vi "Init Communication.vi"(8 "error in (no error)":errorcluster, 10 "Voltage Length":u32, 11 "Item Ref in":T2 format="%.0x") -> (0 "error out":errorcluster, 2 "Communication":T1, 3 "Item Ref out":T2 format="%.0x")   [LabVIEW 2011, in "Switch-DMM Custom Device.lvlib"]
uses:
  Switch-DMM Custom Device.lvlib
  <vilib>/NI Veristand/Custom Device API/Custom Device Item Ref.ctl
  Controls/Communication.ctl
  Controls/Async Status.ctl
  Controls/Async State.ctl
  Controls/Async Command.ctl
  Controls/Async Events.ctl
  <vilib>/NI Veristand/Custom Device API/Custom Device API.lvlib
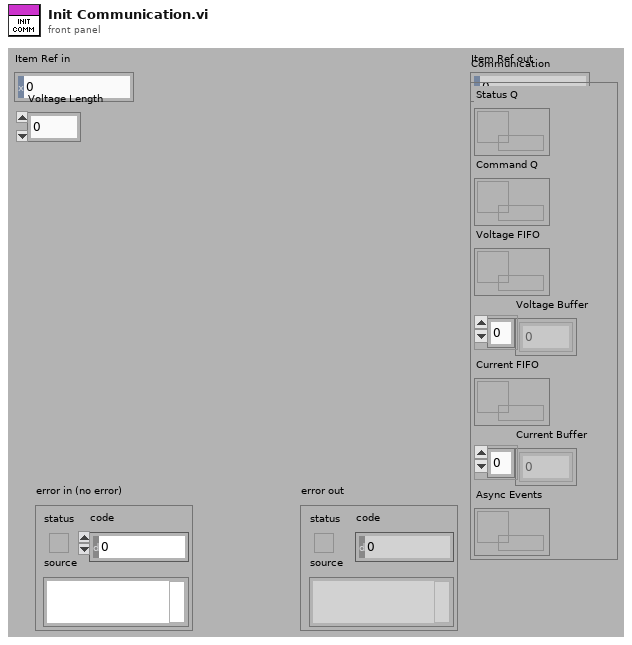
[diagram p1: front panel]
types:
  T1 = typedef "Switch-DMM Custom Device.lvlib/Communication.ctl" = cluster{"Status Q":refnum<queue>, "Command Q":refnum<queue>, "Voltage FIFO":refnum<k33>, "Voltage Buffer":dbl[], "Current FIFO":refnum<k33>, "Current Buffer":dbl[], "Async Events":refnum<queue>}
  T2 = typedef "Custom Device API.lvlib/Custom Device Item Ref.ctl" = u64
  T3 = typedef "Switch-DMM Custom Device.lvlib/Async Events.ctl" = enum16{"None", "Over Current", "Volt Read Done"}
  T4 = typedef "Switch-DMM Custom Device.lvlib/Async Status.ctl" = cluster{"State":T5, "error":errorcluster}
  T5 = typedef "Switch-DMM Custom Device.lvlib/Async State.ctl" = enum16{"Not running", "Initializing", "Waiting on start cmd", "Running", "Stopped"}
  T6 = typedef "Switch-DMM Custom Device.lvlib/Async Command.ctl" = enum16{"None", "Start", "Set Cur Mode", "Req Volt Mode", "Set Volt Mode", "Read Volt", "Exit"}
  T7 = cluster{"read mode":enum16{"polling", "blocking"}, "write mode":enum16{"polling", "blocking"}}
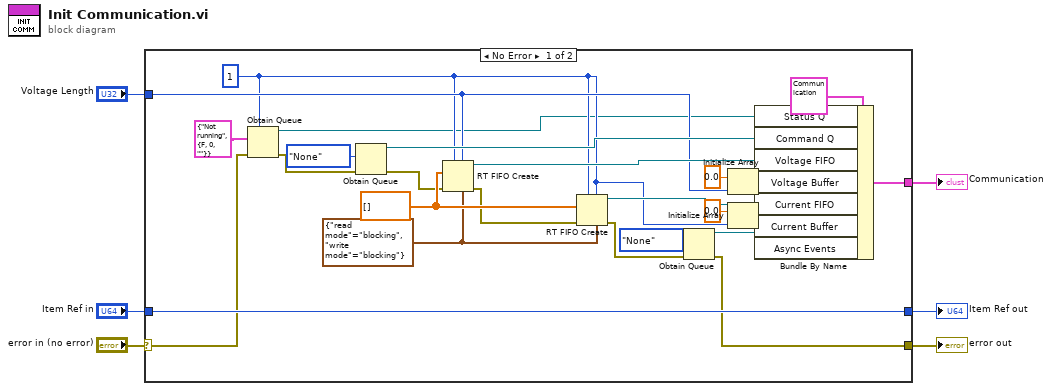
[diagram p0: block diagram]
diagram:
  n1 = case shown="No Error" "error in (no error)" {
    selector: "error in (no error)" -> [w16 w33]
    tunnel: "Item Ref in" -> [w19 w32]
    tunnel: [w7 w33] -> w4
    tunnel: [w19 w32] -> w3
    tunnel: "Voltage Length" -> [w18 _]
    tunnel: [w13 _] -> w1
    frame No Error {
      w24 = T7 {"read mode"=enum."blocking", "write mode"=enum."blocking"} ("r/w modes (polling,polling)")
      w25 = dbl[] []
      w12 = u32 1 ("size (10)")
      n2 = Obtain Queue(max queue size (-1, unlimited)=w12, element data type=T4 {"State"=enum."Not running", "error"={"status"=FALSE, "code"=0, "source"=""}} ("Async Status"), error in (no error)=w16) -> (queue out=w11:refnum<queue>, error out=w17:errorcluster)  [unwired: 2 in, 1 out]
      n3 = Obtain Queue(element data type=Async_Command."None" ("Async Command"), error in (no error)=w17) -> (queue out=w28:refnum<queue>, error out=w15:errorcluster)  [unwired: 3 in, 1 out]
      n4 = RT FIFO Create(1:w25, 3:w15, 4:w12, 6:w18, 7:w24) -> (8:w23:refnum<k33>, 11:w14:errorcluster)  [unwired: 3 in, 1 out]
      n5 = RT FIFO Create(1:w25, 3:w14, 4:w12, 6:w12, 7:w24) -> (8:w22:refnum<k33>, 11:w8:errorcluster)  [unwired: 3 in, 1 out]
      n6 = Obtain Queue(element data type=Async_Events."None" ("Async Events"), error in (no error)=w8) -> (queue out=w9:refnum<queue>, error out=w7:errorcluster)  [unwired: 3 in, 1 out]
      n7 = Initialize Array(0.0, w18) -> (w21:dbl[])
      n8 = Initialize Array(0.0, w12) -> (w20:dbl[])
      n9 = Bundle By Name(cluster=T1 {"Status Q"=refnum, "Command Q"=refnum, "Voltage FIFO"=refnum, "Voltage Buffer"=[], "Current FIFO"=refnum, "Current Buffer"=[], "Async Events"=refnum} ("Communication"), "Status Q"=w11, "Command Q"=w28, "Voltage FIFO"=w23, "Voltage Buffer"=w21, "Current FIFO"=w22, "Current Buffer"=w20, "Async Events"=w9) -> (w13:T1)
    }
    frame Error {
    }
  }
  "error out" <- w4
  "Item Ref out" <- w3
  "Communication" <- w1
